vi "Create.vi"(7 "Available":string[](array[string]), 8 "error in (no error)":errorcluster, 9 "Effective Roles":set{string}(c389), 10 "Current Role":string, 11 "Manager":refnum<class "MessageQ.lvclass">) -> (0 "error out":errorcluster, 3 "Roles API out":refnum<class "Roles API.lvclass">)   [LabVIEW 2020, in "Volatus.lvlib" / "Roles API.lvclass"]
uses:
  Roles API.lvclass
  Roles API.lvclass/Roles API.ctl
  MessageQ/MessageQ.lvclass
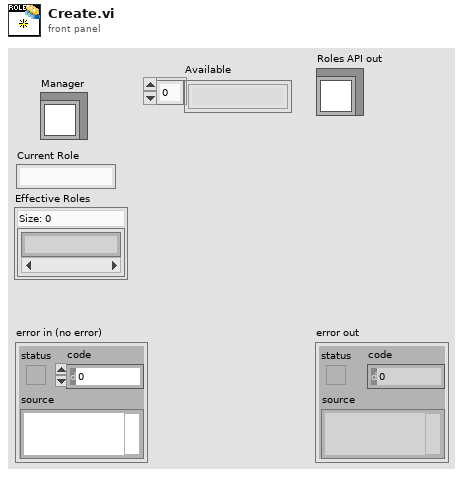
[diagram p1: front panel]
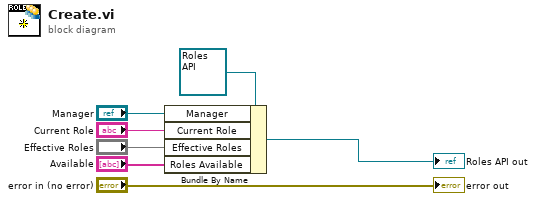
[diagram p0: block diagram]
diagram:
  n1 = Bundle By Name(cluster=refnum<class "Roles API.lvclass"> refnum ("Roles API in"), "Manager"="Manager", "Current Role"="Current Role", "Effective Roles"="Effective Roles", "Roles Available"="Available") -> (→"Roles API out":refnum<class "Roles API.lvclass">)
  "error out" <- "error in (no error)"
